vi "Config Write Arm Globals.vi"(11 "refnum":T1) -> (3 "refnum 2":T1)   [LabVIEW 2012]
uses:
  <vilib>/Utility/config.llb/Config Data RefNum.ctl
  Arm Globals.vi
  <vilib>/Utility/config.llb/Write Key (Double).vi
  <vilib>/Utility/config.llb/NI_LVConfig.lvlib
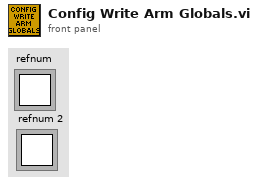
[diagram p1: front panel]
types:
  T1 = typedef "NI_LVConfig.lvlib/Config Data RefNum.ctl" = refnum<k1>
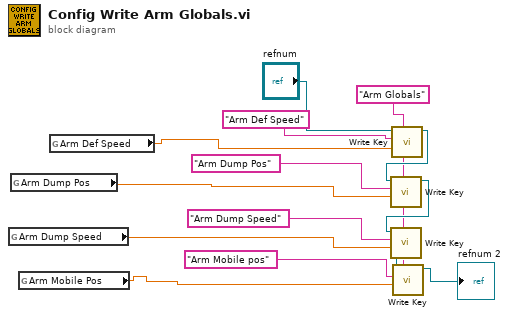
[diagram p0: block diagram]
diagram:
  w6 = "Arm Globals"
  n1 = global read "Arm Globals.vi" "Arm Dump Speed"() -> (w3:dbl)
  n2 = global read "Arm Globals.vi" "Arm Dump Pos"() -> (w2:dbl)
  n3 = global read "Arm Globals.vi" "Arm Mobile Pos"() -> (w4:dbl)
  n4 = global read "Arm Globals.vi" "Arm Def Speed"() -> (w5:dbl)
  n5 = call-poly <vilib>:"Write Key.vi"("section"=w6, "value"=w5, "key"="Arm Def Speed", "refnum"="refnum") -> ("refnum out"=w13:T1)  [unwired: 5 in, 2 out]
  n6 = call-poly <vilib>:"Write Key.vi"("section"=w6, "value"=w2, "key"="Arm Dump Pos", "refnum"=w13) -> ("refnum out"=w12:T1)  [unwired: 5 in, 2 out]
  n7 = call-poly <vilib>:"Write Key.vi"("section"=w6, "value"=w3, "key"="Arm Dump Speed", "refnum"=w12) -> ("refnum out"=w11:T1)  [unwired: 5 in, 2 out]
  n8 = call-poly <vilib>:"Write Key.vi"("section"=w6, "value"=w4, "key"="Arm Mobile pos", "refnum"=w11) -> ("refnum out"=→"refnum 2":T1)  [unwired: 5 in, 2 out]
